vi "Configure OVP.vi"(4 "Channel (3:3)":u16(ring)=1 items=["1"=1, "2"=2, "3"=3], 5 "Channel (2:2)":u16(ring)=1 items=["1"=1, "2"=2, "3"=3], 7 "Channel (1:1)":u16(ring)=1 items=["1"=1, "2"=2, "3"=3], 8 "error in (no error)":errorcluster, 9 "Enable OVP (T: Enable)":bool=TRUE, 10 "Voltage Limit (36.000 V)":dbl=36.0 min=0.0 max=66.0 step=0.001 format="%.3g", 11 "VISA resource name":refnum<visa-resource-name>) -> (0 "error out":errorcluster, 3 "VISA resource name out":refnum<visa-resource-name>)   [LabVIEW 2017, in "BK Precision 913XX.lvlib"]
doc: "Configures over voltage protection (OVP) of the selected channel."
uses:
  <instrlib>/BK Precision 913XX/BK Precision 913XX.lvlib
panel:
  # "V"
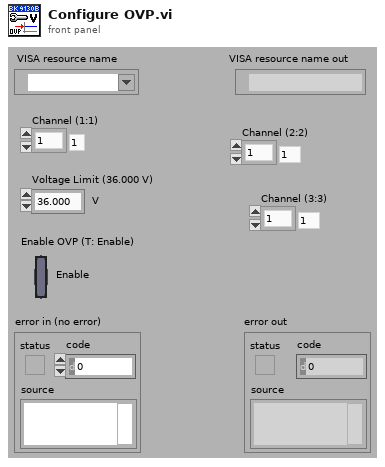
[diagram p1: front panel]
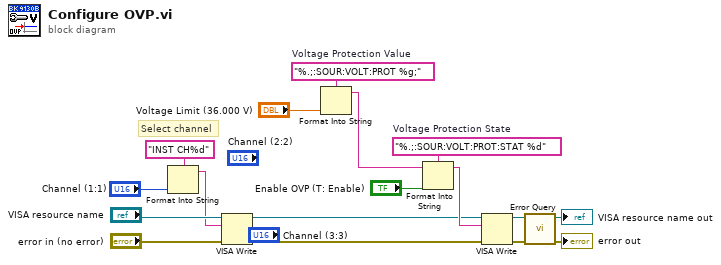
[diagram p0: block diagram]
diagram:
  w14 = "%.;:SOUR:VOLT:PROT:STAT %d"  # Voltage Protection State
  w15 = "%.;:SOUR:VOLT:PROT %g;"  # Voltage Protection Value
  # "Select channel"
  n1 = Format Into String(format string="INST CH%d", "Channel (1:1)") -> (resulting string=w1:string)  [unwired: 2 in, 1 out]
  n2 = VISA Write(VISA resource name="VISA resource name", write buffer=w1, error in (no error)="error in (no error)") -> (VISA resource name out=w4:refnum<visa-resource-name>, error out=w5:errorcluster)  [unwired: 1 out]
  n3 = Format Into String(format string=w15, "Voltage Limit (36.000 V)") -> (resulting string=w8:string)  [unwired: 2 in, 1 out]
  n4 = Format Into String(format string=w14, initial string=w8, "Enable OVP (T: Enable)") -> (resulting string=w13:string)  [unwired: 1 in, 1 out]
  n5 = VISA Write(VISA resource name=w4, write buffer=w13, error in (no error)=w5) -> (VISA resource name out=w11:refnum<visa-resource-name>, error out=w10:errorcluster)  [unwired: 1 out]
  n6 = call <instrlib>:"Error Query.vi"("error in (no error)"=w10, "VISA resource name"=w11) -> ("error out"=→"error out":errorcluster, "VISA resource name out"=→"VISA resource name out":refnum<visa-resource-name>)  [unwired: 6 in, 2 out]
